vi "Untitled 12222.vi"() -> ()   [LabVIEW 2010]
uses:
  <vilib>/NXT/Subs/MotorOutput.ctl
  <vilib>/NXT/Block Support/NXT_InputPort.ctl
  <vilib>/NXT/Dual Mode Library/Motors/MotorOn.vi
  <vilib>/NXT/Dual Mode Library/Waits/Wait_Darkness.vi
  <vilib>/NXT/Dual Mode Library/Waits/Wait_Num.vi
  <vilib>/NXT/Dual Mode Library/Motors/MotorBrake.vi
panel:
  in  "Port (Port 3)":T1=2 items=["Port 1", "Port 2", "Port 3", "Port 4"]
  in  "Power (75)":i32=75
  in  "Output Port (All Ports)":T2=3 items=["Port A", "Port B", "Port C", "All Ports"]
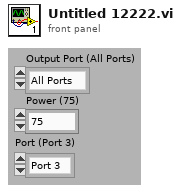
[diagram p1: front panel]
types:
  T1 = typedef "NXT_InputPort.ctl" = u8
  T2 = typedef "MotorOutput.ctl" = u8
  T3 = typedef "LVHSConnector.ctl" = cluster{"error":errorcluster, "address":string, "NXT #":i32, "Show Error":bool, "Connection":u16}
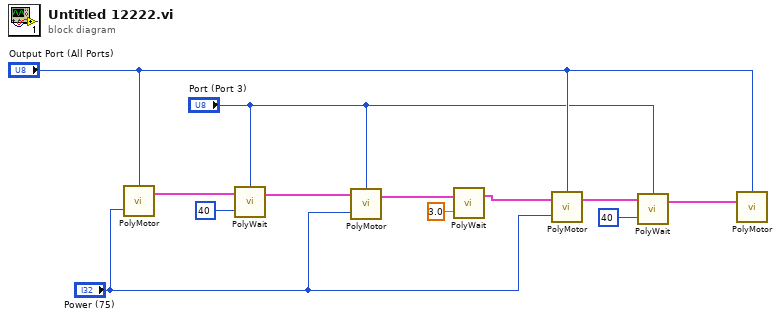
[diagram p0: block diagram]
diagram:
  n1 = call-poly <vilib>:"PolyMotor.vi"("Power (75)"="Power (75)", "Output Port (All Ports)"="Output Port (All Ports)") -> ("NXT"=w12:T3)  [unwired: 2 in]
  n2 = call-poly <vilib>:"PolyWait.vi"("Darkness (40)"=i16 40, "NXT"=w12, "Port (Port 3)"="Port (Port 3)") -> ("NXT"=w11:T3)  [unwired: 1 in]
  n3 = call-poly <vilib>:"PolyMotor.vi"("Power (75)"="Power (75)", "NXT"=w11, "Output Port (All Ports)"="Port (Port 3)") -> ("NXT"=w9:T3)  [unwired: 1 in]
  n4 = call-poly <vilib>:"PolyWait.vi"("Time (sec)"=sgl 3.0, "NXT"=w9) -> ("NXT"=w8:T3)  [unwired: 2 in]
  n5 = call-poly <vilib>:"PolyMotor.vi"("Power (75)"="Power (75)", "NXT"=w8, "Output Port (All Ports)"="Output Port (All Ports)") -> ("NXT"=w7:T3)  [unwired: 1 in]
  n6 = call-poly <vilib>:"PolyWait.vi"("Darkness (40)"=i16 40, "NXT"=w7, "Port (Port 3)"="Port (Port 3)") -> ("NXT"=w6:T3)  [unwired: 1 in]
  n7 = call-poly <vilib>:"PolyMotor.vi"("NXT"=w6, "Port (All Ports)"="Output Port (All Ports)") -> ()  [unwired: 2 in, 1 out]
